vi "outputView.vi"(10 "UserEvents in":refnum<class "UserEvents.lvclass">) -> ()   [LabVIEW 2012]
uses:
  Configuration/Stream Mode Algorithm.ctl
  Typedefs/OutputData.ctl
  UserEvents/UserEvents.lvclass
  Commands/SendOutputData/SendOutputData.lvclass
  UserEvents/UserEvents.lvclass/UserEvents.ctl
  Typedefs/StateSelector.ctl
  Commands/SendOutputData/SendOutputData.lvclass/SendOutputData.ctl
  Commands/SwitchToStreamMode/SwitchToStreamMode.lvclass
  Commands/SwitchToStreamMode/SwitchToStreamMode.lvclass/SwitchToStreamMode.ctl
  Commands/SwitchToOnDemandMode/SwitchToOnDemandMode.lvclass
panel:
  in  "applyIsTrue":bool
  in  "Ch-4":u16(slide) scale=0.0..65535.0
  in  "Ch-3":u16(slide) scale=0.0..65535.0
  in  "Ch-2":u16(slide) scale=0.0..65535.0
  in  "Ch-1":u16(slide) scale=0.0..65535.0
  in  "PWM (SSR)":u8(slide) max=100 scale=0.0..100.0
  in  "Blower RPM":u8(slide) max=127 scale=0.0..127.0
  in  "Step & Direction":i16(slide) min=-128 max=127 scale=-128.0..127.0 scale format="%#.1f"
  out "outputDataIndicator":T1 {"Step & Direction" min=-32767}
  in  "Stream Mode Algorithm":T2
  in  "switchToOnDemandModeIsTrue":bool
  in  "switchToStreamModeIsTrue":bool
  in  "sendIsTrue":bool
  # "DAC"
  # "cts"
  # "cts"
  # "cts"
  # "cts"
  # "(RPM)"
  # "(steps)"
  # "DAC"
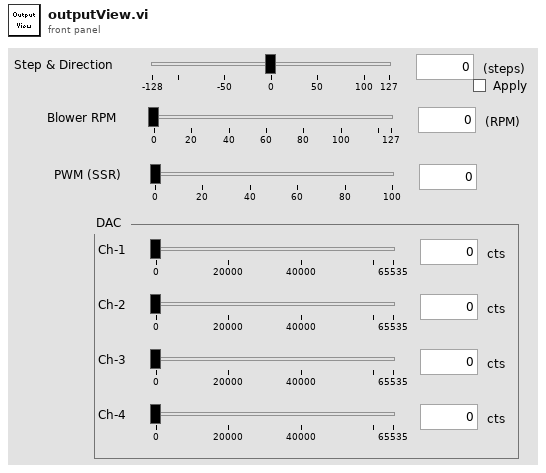
[diagram p1: front panel]
types:
  T1 = typedef "OutputData.ctl" = cluster{"Step & Direction":i16, "Blower RPM":u8, "PWM (SSR)":u8, "Ch1":u16, "Ch2":u16, "Ch3":u16, "Ch4":u16}
  T2 = typedef "Stream Mode Algorithm.ctl" = enum16{"FrontPanelValuesDirectly"}
  T3 = typedef "PubDataEvents.ctl" = cluster{"State":refnum<user-event>, "ErrorCode":refnum<user-event>, "OutputData":refnum<user-event>, "InputData":refnum<user-event>, "ILCConfig":refnum<user-event>, "NeedUserOutputs":refnum<user-event>}
  T4 = typedef "SubDataEvents.ctl" = cluster{"Command":refnum<user-event>}
  T5 = cluster{"Event Registration Refnum":refnum<event-registration>, "Event Registration Refnum":refnum<event-registration>, "Event Registration Refnum":refnum<event-registration>}
  T6 = typedef "StateSelector.ctl" = enum16{"DataOnDemandState", "DataStreamingState", "FaultState", "OffState", "StandbyState"}
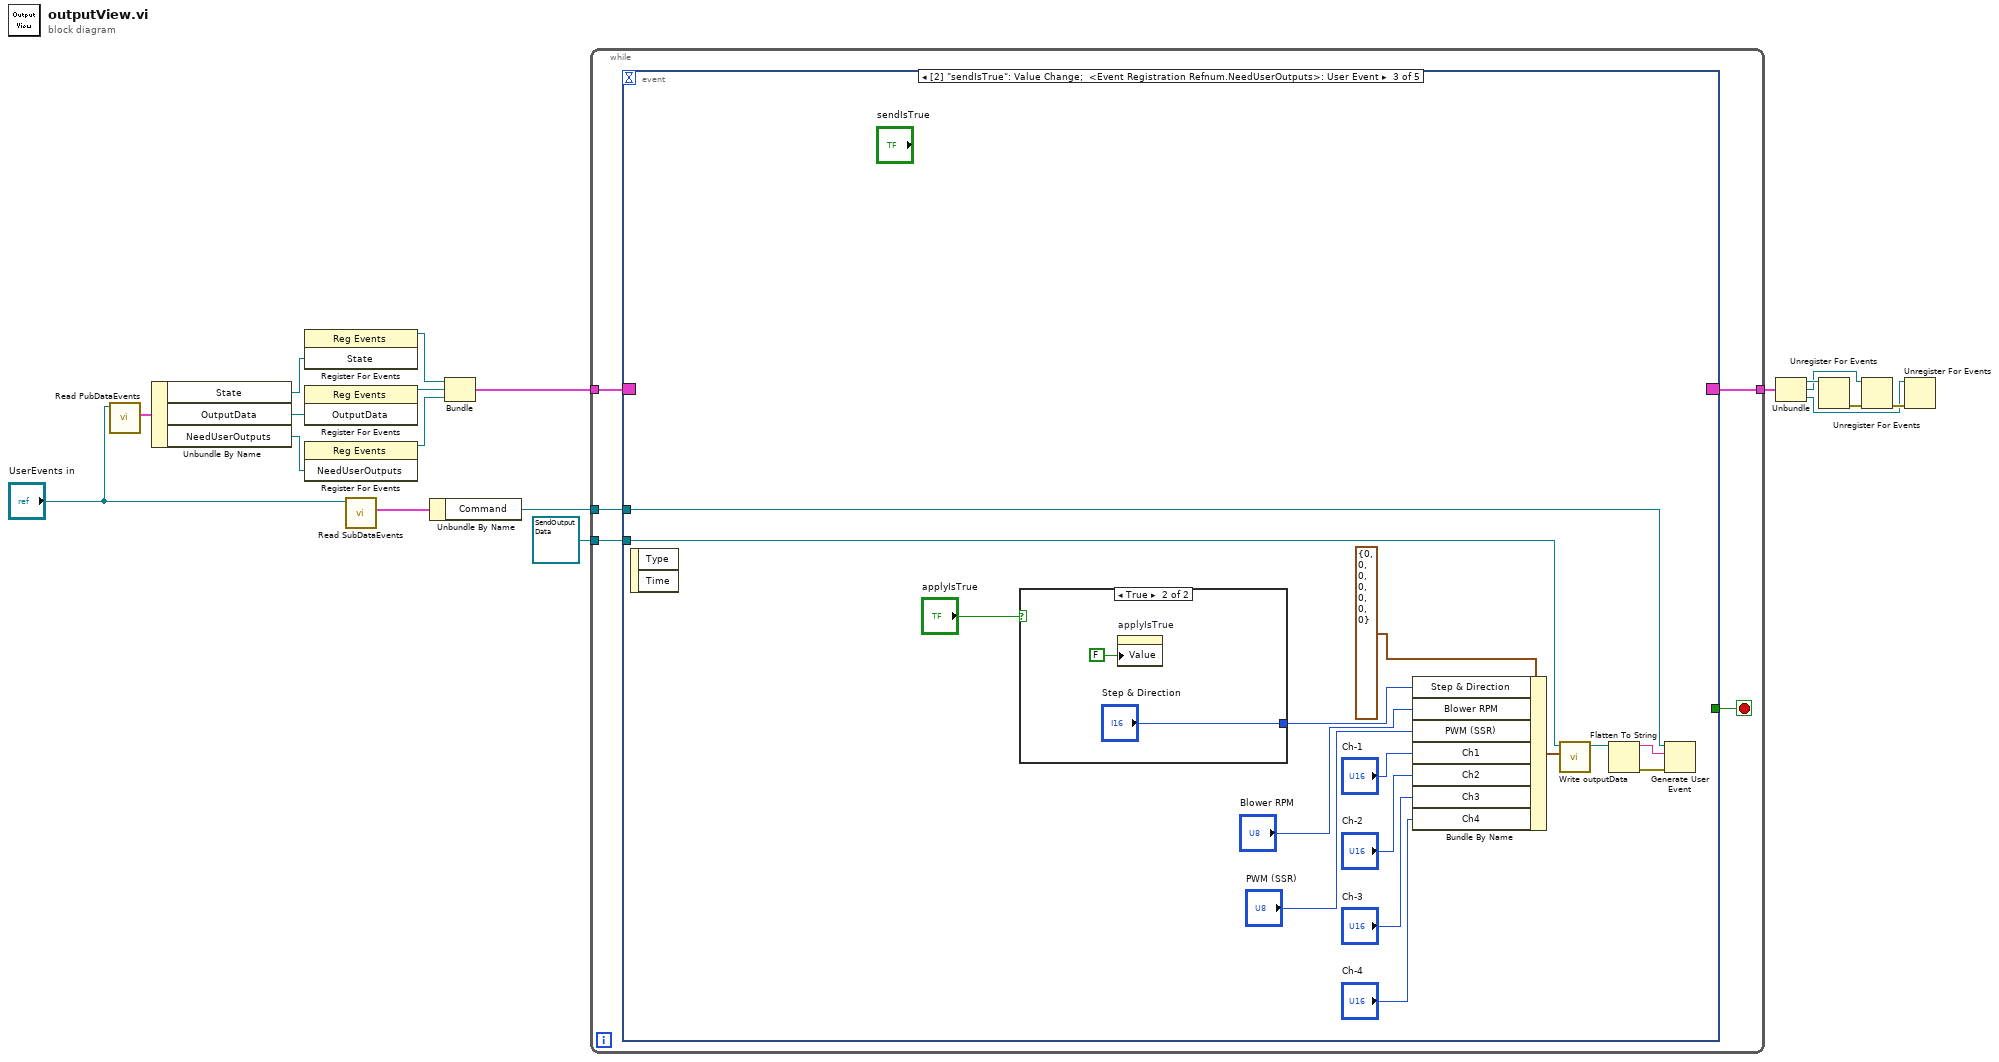
[diagram p0: block diagram]
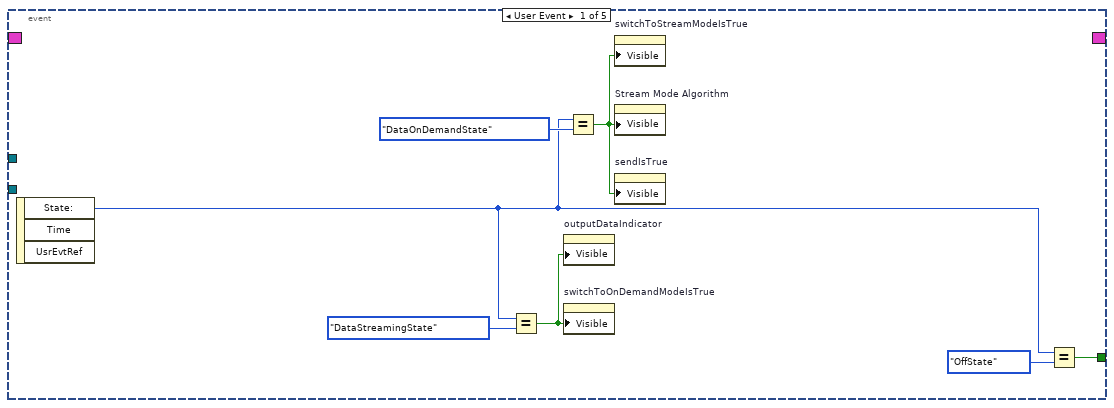
[diagram p2: hidden frame]
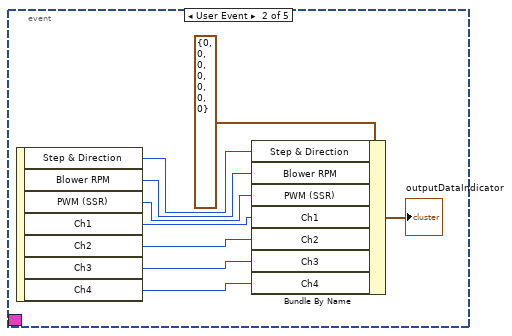
[diagram p3: hidden frame]
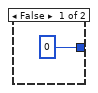
[diagram p4: hidden frame]
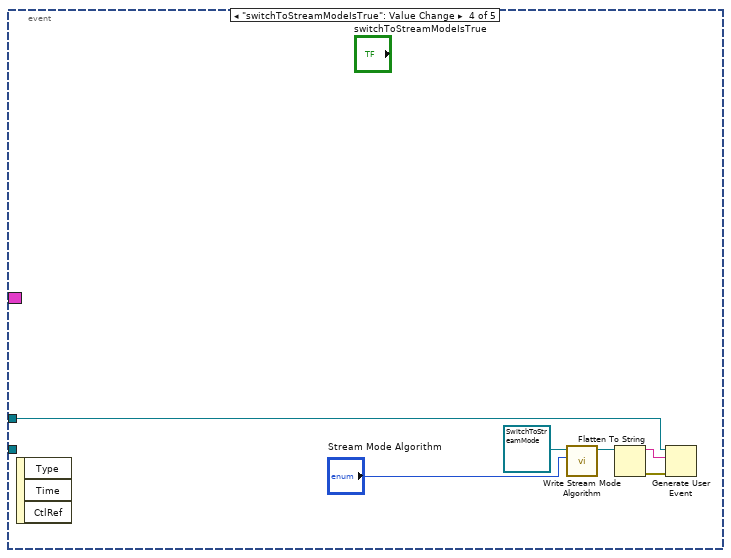
[diagram p5: hidden frame]
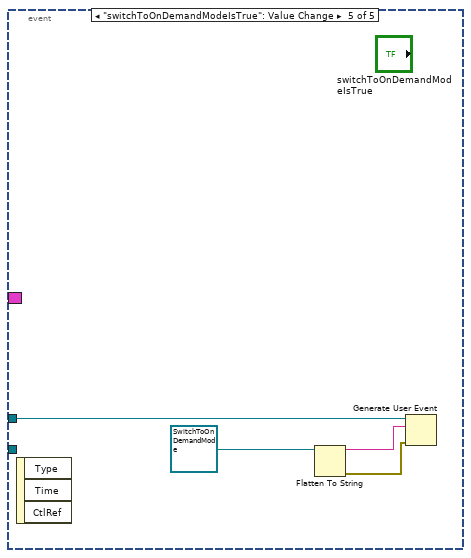
[diagram p6: hidden frame]
diagram:
  n1 = call "Read PubDataEvents.vi"("UserEvents in"="UserEvents in") -> ("PubDataEvents"=w12:T3)  [unwired: 9 in, 1 out]
  n2 = Unbundle By Name(w12) -> ("State"=w14:refnum<user-event>, "OutputData"=w16:refnum<user-event>, "NeedUserOutputs"=w4:refnum<user-event>)
  n3 = register-events(w14) -> (reference out=w15:refnum<event-registration>)  [unwired: 2 in, 1 out]
  n4 = register-events(w16) -> (reference out=w17:refnum<event-registration>)  [unwired: 2 in, 1 out]
  n5 = register-events(w4) -> (reference out=w3:refnum<event-registration>)  [unwired: 2 in, 1 out]
  n6 = call "Read SubDataEvents.vi"("UserEvents in"="UserEvents in") -> ("SubDataEvents"=w13:T4)  [unwired: 9 in, 1 out]
  n7 = Unbundle By Name(w13) -> ("Command"=w10:refnum<user-event>)
  n8 = Bundle("Event Registration Refnum"=w15, "Event Registration Refnum"=w17, "Event Registration Refnum"=w3) -> (w11:T5)  [unwired: 1 in]
  n9 = while {
    tunnel: refnum<class "SendOutputData.lvclass"> refnum ("SendOutputData in") -> [w23]
    tunnel: w11 -> [w22]
    tunnel: w10 -> [w21]
    tunnel: [w20] -> w9
    stop <- w19 stop-if-true
    n10 = event shown="[2] \"sendIsTrue\": Value Change;  <Event Registration Refnum.NeedUserOutputs>: User Event" {
      selector: w22 -> [_ _ _ _ _]
      dyn-events: [_ _ _ _ _] -> w20
      timeout: _ -> [_ _ _ _ _]
      tunnel: w23 -> [_ _ w54 _ _]
      tunnel: w21 -> [_ _ w50 w58 w64]
      tunnel: [w25 _ _ _ _] -> w19
      event User Event {
        n11 = event-data() -> ("State:"=w26:T6)  [unwired: 1 in, 2 out]
        n12 = Equal?(x=w26, y=StateSelector."DataStreamingState") -> (x = y?=w30:bool)
        n13 = property on="outputDataIndicator" class="Clust (strict)"("Visible"=w30) -> ()  [unwired: 2 in, 2 out]
        n14 = property on="switchToOnDemandModeIsTrue" class="Bool"("Visible"=w30) -> ()  [unwired: 2 in, 2 out]
        n15 = Equal?(x=w26, y=StateSelector."DataOnDemandState") -> (x = y?=w24:bool)
        n16 = property on="switchToStreamModeIsTrue" class="Bool"("Visible"=w24) -> ()  [unwired: 2 in, 2 out]
        n17 = property on="Stream Mode Algorithm" class="Enum (strict)"("Visible"=w24) -> ()  [unwired: 2 in, 2 out]
        n18 = property on="sendIsTrue" class="Bool"("Visible"=w24) -> ()  [unwired: 2 in, 2 out]
        n19 = Equal?(x=w26, y=StateSelector."OffState") -> (x = y?=w25:bool)
      }
      event User Event {
        n20 = event-data() -> ("Step & Direction"=w37:i16, "Blower RPM"=w36:u8, "PWM (SSR)"=w35:u8, "Ch1"=w34:u16, "Ch2"=w33:u16, "Ch3"=w32:u16, "Ch4"=w31:u16)  [unwired: 1 in]
        n21 = Bundle By Name(cluster=T1 {"Step & Direction"=0, "Blower RPM"=0, "PWM (SSR)"=0, "Ch1"=0, "Ch2"=0, "Ch3"=0, "Ch4"=0} ("outputDataIndicator"), "Step & Direction"=w37, "Blower RPM"=w36, "PWM (SSR)"=w35, "Ch1"=w34, "Ch2"=w33, "Ch3"=w32, "Ch4"=w31) -> (→"outputDataIndicator":T1)
      }
      event "sendIsTrue": Value Change; User Event {
        n22 = event-data() -> ()  [unwired: 1 in, 2 out]
        n23 = case shown="True" "applyIsTrue" {
          tunnel: [i16 0 ("Step & Direction") "Step & Direction"] -> w47
          frame False {
          }
          frame True {
            n24 = property on="applyIsTrue" class="Bool (strict)"("Value"=FALSE ("applyIsTrue")) -> ()  [unwired: 2 in, 2 out]
          }
        }
        n25 = Bundle By Name(cluster=T1 {"Step & Direction"=0, "Blower RPM"=0, "PWM (SSR)"=0, "Ch1"=0, "Ch2"=0, "Ch3"=0, "Ch4"=0} ("outputDataControl"), "Step & Direction"=w47, "Blower RPM"="Blower RPM", "PWM (SSR)"="PWM (SSR)", "Ch1"="Ch-1", "Ch2"="Ch-2", "Ch3"="Ch-3", "Ch4"="Ch-4") -> (w48:T1)
        n26 = call "Write outputData.vi"("outputData"=w48, "SendOutputData in"=w54) -> ("SendOutputData out"=w53:refnum<class "SendOutputData.lvclass">)  [unwired: 9 in]
        n27 = Flatten To String(anything=w53) -> (data string=w52:string, error out=w51:errorcluster)  [unwired: 3 in, 1 out]
        n28 = Generate User Event(user event=w50, event data cluster=w52, error in=w51) -> ()  [unwired: 2 out]
      }
      event "switchToStreamModeIsTrue": Value Change {
        n29 = event-data() -> ()  [unwired: 1 in, 3 out]
        n30 = call "Write Stream Mode Algorithm.vi"("Stream Mode Algorithm"="Stream Mode Algorithm", "SwitchToStreamMode in"=refnum<class "SwitchToStreamMode.lvclass"> refnum ("SwitchToStreamMode.lvclass")) -> ("SwitchToStreamMode out"=w62:refnum<class "SwitchToStreamMode.lvclass">)  [unwired: 9 in]
        n31 = Flatten To String(anything=w62) -> (data string=w60:string, error out=w59:errorcluster)  [unwired: 3 in, 1 out]
        n32 = Generate User Event(user event=w58, event data cluster=w60, error in=w59) -> ()  [unwired: 2 out]
      }
      event "switchToOnDemandModeIsTrue": Value Change {
        n33 = event-data() -> ()  [unwired: 1 in, 3 out]
        n34 = Flatten To String(anything=refnum<class "SwitchToOnDemandMode.lvclass"> refnum ("SwitchToOnDemandMode.lvclass")) -> (data string=w66:string, error out=w65:errorcluster)  [unwired: 3 in, 1 out]
        n35 = Generate User Event(user event=w64, event data cluster=w66, error in=w65) -> ()  [unwired: 2 out]
      }
    }
  }
  n36 = Unbundle(w9) -> ("Event Registration Refnum"=w8:refnum<event-registration>, "Event Registration Refnum"=w6:refnum<event-registration>, "Event Registration Refnum"=w1:refnum<event-registration>)
  n37 = Unregister For Events(event registration refnum=w8) -> (error out=w7:errorcluster)  [unwired: 1 in]
  n38 = Unregister For Events(event registration refnum=w6, error in=w7) -> (error out=w2:errorcluster)
  n39 = Unregister For Events(event registration refnum=w1, error in=w2) -> ()  [unwired: 1 out]
